vi "Loop_ACT_Drive with Profile.vi"() -> ()   [LabVIEW 2017]
uses:
  _SHARE ALL/Global Share All/Global_STOP.vi
  Global_ACT Write_Data Out.vi
  Global_SM Write_Data Out.vi
  WCDrive2018/WCDrive2018.lvlib
  TypeDef/CLUSTER_Drive_HW_SRX_Status.ctl
  TypeDef/ENUM_Drive_ACT Loop_Mode.ctl
  TypeDef/CLUSTER_X and Y.ctl
  TypeDef/ENUM_Drive_Profile_CMD.ctl
  Dashboard/Global_SEN Write_Data.vi
  TypeDef/CLUSTER_Drive_Point Specification.ctl
  TypeDef/CLUSTER_Drive_Motion Profile Arrays.ctl
  TypeDef/CLUSTER_SRX_Profile Data.ctl
  TypeDef/CLUSTER_SRX_Limit Switch Data.ctl
  TypeDef/CLUSTER_SRX_Analog Data.ctl
  TypeDef/CLUSTER_SRX_PWM Data.ctl
  TypeDef/CLUSTER_SRX_Encoder Data.ctl
  TypeDef/CLUSTER_SRX_Status Data.ctl
  TypeDef/CLUSTER_4296_SRX_Status.ctl
  TypeDef/ENUM_Drive_SRX Motion Buffer Status.ctl
panel:
  out "Output Data":dbl
  out "Input Data":dbl
  out "Cycle Time (S)":dbl format="%.3g"
  in  "Target Time(ms)":u32=50
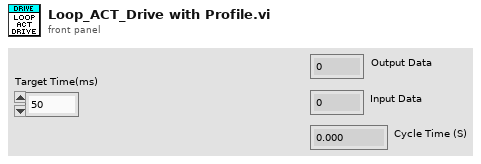
[diagram p1: front panel]
types:
  T1 = typedef "ENUM_Drive_SRX Motion Buffer Status.ctl" = cluster{"Index":i32, "Last Point":bool}
  T2 = typedef "CLUSTER_Drive_Motion Profile Arrays.ctl" = cluster{"Left":T3[], "Right":T3[]}
  T3 = typedef "CLUSTER_Drive_Point Specification.ctl" = cluster{"Position":dbl, "Velocity":dbl, "headingDeg":dbl, "Duration in ms":i32}
  T4 = typedef "ENUM_Drive_Profile_CMD.ctl" = enum16{"Stop", "Setup", "Run"}
  T5 = typedef "CLUSTER_X and Y.ctl" = cluster{"Steer":dbl, "Throtle":dbl}
  T6 = typedef "ENUM_Drive_ACT Loop_Mode.ctl" = enum16{"Stop", "Position", "VBus", "Profile"}
  T7 = typedef "CLUSTER_Drive_HW_SRX_Status.ctl" = cluster{"Rear Left":T8, "Rear Right":T8, "Front Left":T8, "Front Right":T8}
  T8 = typedef "CLUSTER_4296_SRX_Status.ctl" = cluster{"Status":T9, "Encoder":T10, "PWM ":T11, "Analog":T12, "Limit Switches":T13, "Profile":T14}
  T9 = typedef "CLUSTER_SRX_Status Data.ctl" = cluster{"Module Enabled":bool, "Current Profile Slot Select":dbl, "Brake is Enabled":bool, "Applied Throttle":dbl, "Current":dbl, "Battery Voltage":dbl, "Sticky Fault - Under Voltage":bool, "Temperature (C)":dbl, "Sticky Fault - Over Temp":bool, "CAN Error":errorcluster, "Control 5 Is Supported":bool}
  T10 = typedef "CLUSTER_SRX_Encoder Data.ctl" = cluster{"Closed Loop Error":dbl, "Sensor Position":dbl, "Sensor Velocity":dbl, "Encoder Position":dbl, "Encoder Velocity":dbl, "Encoder Index Count":dbl, "Encoder A Pin State":bool, "Encoder B Pin State":bool, "Encoder Index Pin State":bool, "Pos Div 8":bool, "Vel Div 4":bool}
  T11 = typedef "CLUSTER_SRX_PWM Data.ctl" = cluster{"Closed Loop Error":dbl, "Pulse Width Position":i32, "Pulse Width Velocity":i32, "Pulse Width Rise To Rise (us)":i32, "Pulse Width Rise To Fall (us)":i32}
  T12 = typedef "CLUSTER_SRX_Analog Data.ctl" = cluster{"Closed Loop Error":dbl, "Analog In":dbl, "Analog In Velocity":dbl}
  T13 = typedef "CLUSTER_SRX_Limit Switch Data.ctl" = cluster{"Forward Limit Switch Closed":bool, "Reverse Limit Switch Closed":bool, "Sticky Fault - Forward Limit":bool, "Sticky Fault - Reverse Limit":bool, "Sticky Fault - Forward Soft Limit":bool, "Sticky Fault - Reverse Soft Limit":bool}
  T14 = typedef "CLUSTER_SRX_Profile Data.ctl" = cluster{"Mot Prof Active Is Under Run":bool, "Mot Prof Active Has Under Run":bool, "Mot Prof Active Is Last":bool, "Mot Prof Active Velocity Only":bool, "Mot Prof Active Is Valid":bool, "Mot Prof Buffer Is Full":bool, "Mot Prof Active Profile Slot Select":i32, "Mot Prof NextID":i32, "Mot Prof Count":i32, "Mot Prof Active Velocity":dbl, "Mot Prof Active Position":dbl, "Mot Prof Output Enable":i32}
  T15 = typedef "WPI_RobotDriveDevRef.ctl" = cluster{"DevStatus":errorcluster, "Motors[]":T16[], "Square Inputs":bool, "Max Output":dbl}
  T16 = typedef "WPI_MotorControlDeviceRef.ctl" = cluster{"DeviceStatus":errorcluster, "Type":T17, "PWM":cluster{"PWM Channel":T18, "DeadBand":T19}, "CAN":cluster{"Device Number":u8, "SetOutput VI Ref":variant, "GetOutput VI Ref":variant, "Enable VI Ref":variant, "Disable VI Ref":variant, "Data":variant}, "Invert":bool, "DIO PWM":cluster{"PWM \"Enable\" Channel":T18, "DIOChannel":T20, "PWM Rate":dbl}}
  T17 = typedef "WPI_MotorControlType.ctl" = enum16{"PWM", "CAN", "DIO PWM"}
  T18 = typedef "FPGA_DIOPWMChannel.ctl" = enum8{"PWM 0", "PWM 1", "PWM 2", "PWM 3", "PWM 4", "PWM 5", "PWM 6", "PWM 7", "PWM 8", "PWM 9", "PWM MXP 0", "PWM MXP 1", "PWM MXP 2", "PWM MXP 3", "PWM MXP 4", "PWM MXP 5", "PWM MXP 6", "PWM MXP 7", "PWM MXP 8", "PWM MXP 9", "Invalid"}
  T19 = typedef "WPI_PWMDeadband.ctl" = cluster{"Name":string, "maxPositivePwm":i32, "minPositivePwm":i32, "centerPwm":i32, "maxNegativePwm":i32, "minNegativePwm":i32, "angularRange":u16}
  T20 = typedef "FPGA_DIOChannel.ctl" = enum8{"DIO 0", "DIO 1", "DIO 2", "DIO 3", "DIO 4", "DIO 5", "DIO 6", "DIO 7", "DIO 8", "DIO 9", "DIO MXP 0", "DIO MXP 1", "DIO MXP 2", "DIO MXP 3", "DIO MXP 4", "DIO MXP 5", "DIO MXP 6", "DIO MXP 7", "DIO MXP 8", "DIO MXP 9", "DIO MXP 10", "DIO MXP 11", "DIO MXP 12", "DIO MXP 13", "DIO MXP 14", "DIO MXP 15", "SPI Port CS1", "SPI Port CS2", "SPI Port CS3", "SPI Port MISO", "SPI Port MOSI", "Invalid"}
  T21 = cluster{"RobotDriveDevRef Out":T15, "Target Time(ms)":u32, "Current Time":timestamp, "Previous Time":timestamp, "Cycle Time (S)":dbl, "SRX_Status":T7, "Mode":T6, "VBus":T5, "ProfileCmd":T4, "MotionProfiles":T2, "Buffer Status Array":T1[]}
  T22 = typedef "CLUSTER_Left and Right.ctl" = cluster{"Left":dbl, "Right":dbl}
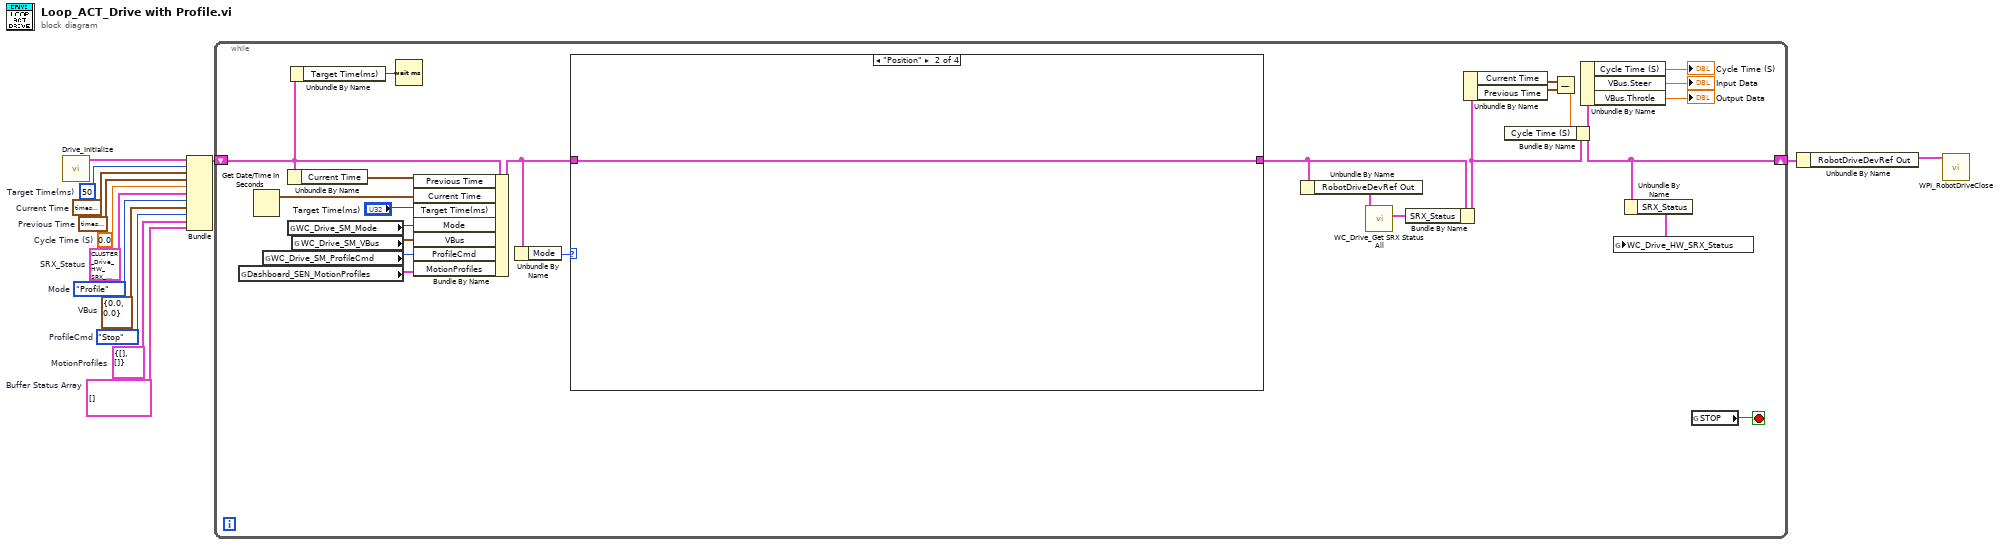
[diagram p0: block diagram]
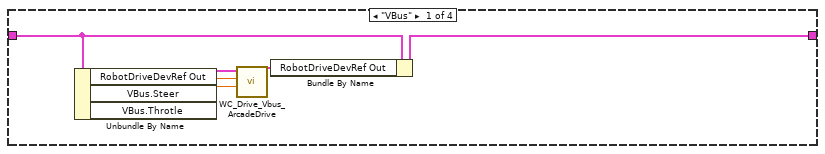
[diagram p2: hidden frame]
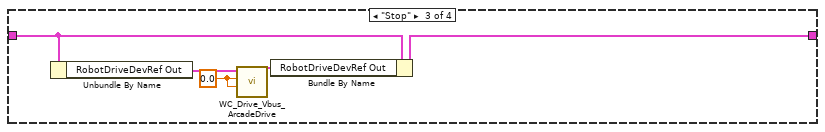
[diagram p3: hidden frame]
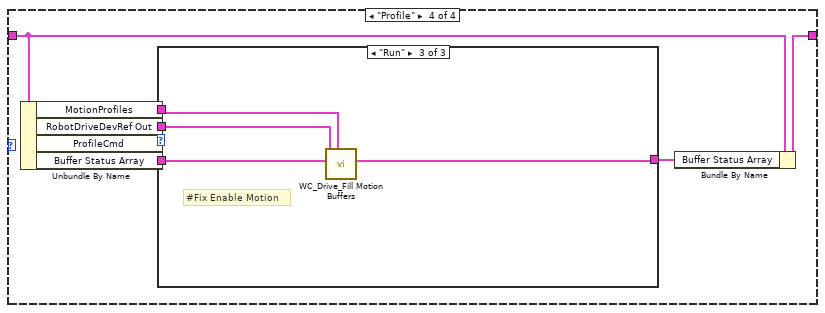
[diagram p4: hidden frame]
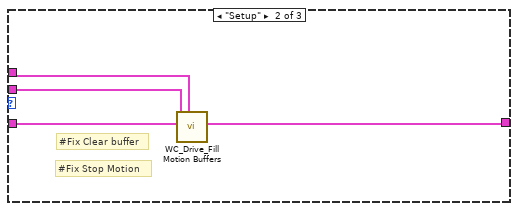
[diagram p6: hidden frame]
diagram:
  w1 = T1[] []  # Buffer Status Array
  w2 = T2 {"Left"=[], "Right"=[]}  # MotionProfiles
  w3 = ENUM_Drive_Profile_CMD."Stop"  # ProfileCmd
  w4 = T5 {"Steer"=0.0, "Throtle"=0.0}  # VBus
  w5 = ENUM_Drive_ACT_Loop_Mode."Profile"  # Mode
  w6 = T7 {"Rear Left"={"Status"={"Module Enabled"=FALSE, "Current Profile Slot Select"=0.0, "Brake is Enabled"=FALSE, "Applied Throttle"=0.0, "Current"=0.0, "Battery Voltage"=0.0, "Sticky Fault - Under Voltage"=FALSE, "Temperature (C)"=0.0, "Sticky Fault - Over Temp"=FALSE, "CAN Error"={"status"=FALSE, "code"=0, "source"=""}, "Control 5 Is Supported"=FALSE}, "Encoder"={"Closed Loop Error"=0.0, "Sensor Position"=0.0, "Sensor Velocity"=0.0, "Encoder Position"=0.0, "Encoder Velocity"=0.0, "Encoder Index Count"=0.0, "Encoder A Pin State"=FALSE, "Encoder B Pin State"=FALSE, "Encoder Index Pin State"=FALSE, "Pos Div 8"=FALSE, "Vel Div 4"=FALSE}, "PWM "={"Closed Loop Error"=0.0, "Pulse Width Position"=0, "Pulse Width Velocity"=0, "Pulse Width Rise To Rise (us)"=0, "Pulse Width Rise To Fall (us)"=0}, "Analog"={"Closed Loop Error"=0.0, "Analog In"=0.0, "Analog In Velocity"=0.0}, "Limit Switches"={"Forward Limit Switch Closed"=FALSE, "Reverse Limit Switch Closed"=FALSE, "Sticky Fault - Forward Limit"=FALSE, "Sticky Fault - Reverse Limit"=FALSE, "Sticky Fault - Forward Soft Limit"=FALSE, "Sticky Fault - Reverse Soft Limit"=FALSE}, "Profile"={"Mot Prof Active Is Under Run"=FALSE, "Mot Prof Active Has Under Run"=FALSE, "Mot Prof Active Is Last"=FALSE, "Mot Prof Active Velocity Only"=FALSE, "Mot Prof Active Is Valid"=FALSE, "Mot Prof Buffer Is Full"=FALSE, "Mot Prof Active Profile Slot Select"=0, "Mot Prof NextID"=0, "Mot Prof Count"=0, "Mot Prof Active Velocity"=0.0, "Mot Prof Active Position"=0.0, "Mot Prof Output Enable"=0}}, "Rear Right"={"Status"={"Module Enabled"=FALSE, "Current Profile Slot Select"=0.0, "Brake is Enabled"=FALSE, "Applied Throttle"=0.0, "Current"=0.0, "Battery Voltage"=0.0, "Sticky Fault - Under Voltage"=FALSE, "Temperature (C)"=0.0, "Sticky Fault - Over Temp"=FALSE, "CAN Error"={"status"=FALSE, "code"=0, "source"=""}, "Control 5 Is Supported"=FALSE}, "Encoder"={"Closed Loop Error"=0.0, "Sensor Position"=0.0, "Sensor Velocity"=0.0, "Encoder Position"=0.0, "Encoder Velocity"=0.0, "Encoder Index Count"=0.0, "Encoder A Pin State"=FALSE, "Encoder B Pin State"=FALSE, "Encoder Index Pin State"=FALSE, "Pos Div 8"=FALSE, "Vel Div 4"=FALSE}, "PWM "={"Closed Loop Error"=0.0, "Pulse Width Position"=0, "Pulse Width Velocity"=0, "Pulse Width Rise To Rise (us)"=0, "Pulse Width Rise To Fall (us)"=0}, "Analog"={"Closed Loop Error"=0.0, "Analog In"=0.0, "Analog In Velocity"=0.0}, "Limit Switches"={"Forward Limit Switch Closed"=FALSE, "Reverse Limit Switch Closed"=FALSE, "Sticky Fault - Forward Limit"=FALSE, "Sticky Fault - Reverse Limit"=FALSE, "Sticky Fault - Forward Soft Limit"=FALSE, "Sticky Fault - Reverse Soft Limit"=FALSE}, "Profile"={"Mot Prof Active Is Under Run"=FALSE, "Mot Prof Active Has Under Run"=FALSE, "Mot Prof Active Is Last"=FALSE, "Mot Prof Active Velocity Only"=FALSE, "Mot Prof Active Is Valid"=FALSE, "Mot Prof Buffer Is Full"=FALSE, "Mot Prof Active Profile Slot Select"=0, "Mot Prof NextID"=0, "Mot Prof Count"=0, "Mot Prof Active Velocity"=0.0, "Mot Prof Active Position"=0.0, "Mot Prof Output Enable"=0}}, "Front Left"={"Status"={"Module Enabled"=FALSE, "Current Profile Slot Select"=0.0, "Brake is Enabled"=FALSE, "Applied Throttle"=0.0, "Current"=0.0, "Battery Voltage"=0.0, "Sticky Fault - Under Voltage"=FALSE, "Temperature (C)"=0.0, "Sticky Fault - Over Temp"=FALSE, "CAN Error"={"status"=FALSE, "code"=0, "source"=""}, "Control 5 Is Supported"=FALSE}, "Encoder"={"Closed Loop Error"=0.0, "Sensor Position"=0.0, "Sensor Velocity"=0.0, "Encoder Position"=0.0, "Encoder Velocity"=0.0, "Encoder Index Count"=0.0, "Encoder A Pin State"=FALSE, "Encoder B Pin State"=FALSE, "Encoder Index Pin State"=FALSE, "Pos Div 8"=FALSE, "Vel Div 4"=FALSE}, "PWM "={"Closed Loop Error"=0.0, "Pulse Width Position"=0, "Pulse Width Velocity"=0, "Pulse Width Rise To Rise (us)"=0, "Pulse Width Rise To Fall (us)"=0}, "Analog"={"Closed Loop Error"=0.0, "Analog In"=0.0, "Analog In Velocity"=0.0}, "Limit Switches"={"Forward Limit Switch Closed"=FALSE, "Reverse Limit Switch Closed"=FALSE, "Sticky Fault - Forward Limit"=FALSE, "Sticky Fault - Reverse Limit"=FALSE, "Sticky Fault - Forward Soft Limit"=FALSE, "Sticky Fault - Reverse Soft Limit"=FALSE}, "Profile"={"Mot Prof Active Is Under Run"=FALSE, "Mot Prof Active Has Under Run"=FALSE, "Mot Prof Active Is Last"=FALSE, "Mot Prof Active Velocity Only"=FALSE, "Mot Prof Active Is Valid"=FALSE, "Mot Prof Buffer Is Full"=FALSE, "Mot Prof Active Profile Slot Select"=0, "Mot Prof NextID"=0, "Mot Prof Count"=0, "Mot Prof Active Velocity"=0.0, "Mot Prof Active Position"=0.0, "Mot Prof Output Enable"=0}}, "Front Right"={"Status"={"Module Enabled"=FALSE, "Current Profile Slot Select"=0.0, "Brake is Enabled"=FALSE, "Applied Throttle"=0.0, "Current"=0.0, "Battery Voltage"=0.0, "Sticky Fault - Under Voltage"=FALSE, "Temperature (C)"=0.0, "Sticky Fault - Over Temp"=FALSE, "CAN Error"={"status"=FALSE, "code"=0, "source"=""}, "Control 5 Is Supported"=FALSE}, "Encoder"={"Closed Loop Error"=0.0, "Sensor Position"=0.0, "Sensor Velocity"=0.0, "Encoder Position"=0.0, "Encoder Velocity"=0.0, "Encoder Index Count"=0.0, "Encoder A Pin State"=FALSE, "Encoder B Pin State"=FALSE, "Encoder Index Pin State"=FALSE, "Pos Div 8"=FALSE, "Vel Div 4"=FALSE}, "PWM "={"Closed Loop Error"=0.0, "Pulse Width Position"=0, "Pulse Width Velocity"=0, "Pulse Width Rise To Rise (us)"=0, "Pulse Width Rise To Fall (us)"=0}, "Analog"={"Closed Loop Error"=0.0, "Analog In"=0.0, "Analog In Velocity"=0.0}, "Limit Switches"={"Forward Limit Switch Closed"=FALSE, "Reverse Limit Switch Closed"=FALSE, "Sticky Fault - Forward Limit"=FALSE, "Sticky Fault - Reverse Limit"=FALSE, "Sticky Fault - Forward Soft Limit"=FALSE, "Sticky Fault - Reverse Soft Limit"=FALSE}, "Profile"={"Mot Prof Active Is Under Run"=FALSE, "Mot Prof Active Has Under Run"=FALSE, "Mot Prof Active Is Last"=FALSE, "Mot Prof Active Velocity Only"=FALSE, "Mot Prof Active Is Valid"=FALSE, "Mot Prof Buffer Is Full"=FALSE, "Mot Prof Active Profile Slot Select"=0, "Mot Prof NextID"=0, "Mot Prof Count"=0, "Mot Prof Active Velocity"=0.0, "Mot Prof Active Position"=0.0, "Mot Prof Output Enable"=0}}}  # SRX_Status
  w9 = 0.0  # Cycle Time (S)
  w14 = timestamp(0 s since 1904-01-01)  # Previous Time
  w13 = timestamp(0 s since 1904-01-01)  # Current Time
  w12 = u32 50  # Target Time(ms)
  n1 = call "Drive_Initialize.vi"() -> ("RobotDriveDevRef Out"=w8:T15)  [unwired: 11 in]
  n2 = Bundle("RobotDriveDevRef Out"=w8, "Target Time(ms)"=w12, "Current Time"=w13, "Previous Time"=w14, "Cycle Time (S)"=w9, "SRX_Status"=w6, "Mode"=w5, "VBus"=w4, "ProfileCmd"=w3, "MotionProfiles"=w2, "Buffer Status Array"=w1) -> (w11:T21)  [unwired: 1 in]
  n3 = while {
    shift-right: [w22] -> w10
    shift-left: w11 -> [w18]
    stop <- w38 stop-if-true
    n4 = global read "Global_SEN Write_Data.vi" "Dashboard_SEN_MotionProfiles"() -> (w16:T2)
    n5 = Get Date/Time In Seconds() -> (seconds since 1Jan1904=w37:timestamp)
    n6 = global read "Global_SM Write_Data Out.vi" "WC_Drive_SM_ProfileCmd"() -> (w19:T4)
    n7 = Unbundle By Name(w18) -> ("Current Time"=w36:timestamp)
    n8 = global read "Global_SM Write_Data Out.vi" "WC_Drive_SM_Mode"() -> (w27:T6)
    n9 = Unbundle By Name(w18) -> ("Target Time(ms)"=w32:u32)
    n10 = global read "Global_SM Write_Data Out.vi" "WC_Drive_SM_VBus"() -> (w26:T22)
    n11 = Wait (ms)(milliseconds to wait=w32) -> ()  [unwired: 1 out]
    n12 = Bundle By Name(cluster=w18, "Previous Time"=w36, "Current Time"=w37, "Target Time(ms)"="Target Time(ms)", "Mode"=w27, "VBus"=w26, "ProfileCmd"=w19, "MotionProfiles"=w16) -> (w25:T21)
    n13 = Unbundle By Name(w25) -> ("Mode"=w24:T6)
    n14 = case shown="\"Position\"" w24 {
      tunnel: w25 -> [w40 w45 w48 w53]
      tunnel: [w39 w45 w47 w52] -> w20
      frame "VBus" {
        n15 = Unbundle By Name(w40) -> ("RobotDriveDevRef Out"=w44:T15, "VBus.Steer"=w43:dbl, "VBus.Throtle"=w42:dbl)
        n16 = call "WC_Drive_Vbus_ArcadeDrive.vi"("Right Value"=w42, "Left Value"=w43, "RobotDriveDevRef"=w44) -> ("RobotDriveDevRef Out"=w41:T15)  [unwired: 7 in, 1 out]
        n17 = Bundle By Name(cluster=w40, "RobotDriveDevRef Out"=w41) -> (w39:T21)
      }
      frame "Position" {
      }
      frame "Stop" {
        w46 = 0.0 ("X axis value")
        n18 = Unbundle By Name(w48) -> ("RobotDriveDevRef Out"=w50:T15)
        n19 = call "WC_Drive_Vbus_ArcadeDrive.vi"("Right Value"=w46, "Left Value"=w46, "RobotDriveDevRef"=w50) -> ("RobotDriveDevRef Out"=w49:T15)  [unwired: 7 in, 1 out]
        n20 = Bundle By Name(cluster=w48, "RobotDriveDevRef Out"=w49) -> (w47:T21)
      }
      frame "Profile" {
        n21 = Unbundle By Name(w53) -> ("MotionProfiles"=w55:T2, "RobotDriveDevRef Out"=w56:T15, "ProfileCmd"=w57:T4, "Buffer Status Array"=w54:T1[])
        n22 = case shown="\"Run\"" w57 {
          tunnel: w56 -> [_ w59 w63]
          tunnel: w55 -> [_ w60 w64]
          tunnel: w54 -> [w58 w62 w66]
          tunnel: [w58 w61 w65] -> w51
          frame "Stop" {
            # "#Fix Disable Motion"
          }
          frame "Setup" {
            # "#Fix Stop Motion"
            # "#Fix Clear buffer"
            n23 = call "WC_Drive_Fill Motion Buffers.vi"("MotionProfiles"=w60, "Buffer Status Array"=w62, "RobotDriveDevRef"=w59) -> ("Buffer Status Array Out"=w61:T1[])  [unwired: 5 in, 3 out]
          }
          frame "Run" {
            # "#Fix Enable Motion"
            n24 = call "WC_Drive_Fill Motion Buffers.vi"("MotionProfiles"=w64, "Buffer Status Array"=w66, "RobotDriveDevRef"=w63) -> ("Buffer Status Array Out"=w65:T1[])  [unwired: 5 in, 3 out]
          }
        }
        n25 = Bundle By Name(cluster=w53, "Buffer Status Array"=w51) -> (w52:T21)
      }
    }
    n26 = Unbundle By Name(w20) -> ("RobotDriveDevRef Out"=w17:T15)
    n27 = call "WC_Drive_Get SRX Status All.vi"("WC DevRef"=w17) -> ("WC_Drive_SRX Status Out"=w15:T7)  [unwired: 8 in, 2 out]
    n28 = Bundle By Name(cluster=w20, "SRX_Status"=w15) -> (w21:T21)
    n29 = Unbundle By Name(w21) -> ("Current Time"=w35:timestamp, "Previous Time"=w34:timestamp)
    n30 = Subtract(x=w35, y=w34) -> (x-y=w23:dbl)
    n31 = Bundle By Name(cluster=w21, "Cycle Time (S)"=w23) -> (w22:T21)
    n32 = Unbundle By Name(w22) -> ("Cycle Time (S)"=→"Cycle Time (S)":dbl, "VBus.Steer"=→"Input Data":dbl, "VBus.Throtle"=→"Output Data":dbl)
    n33 = Unbundle By Name(w22) -> ("SRX_Status"=w28:T7)
    n34 = global write "Global_ACT Write_Data Out.vi" "WC_Drive_HW_SRX_Status"(w28) -> ()
    n35 = global read "Global_STOP.vi" "STOP"() -> (w38:bool)
  }
  n36 = Unbundle By Name(w10) -> ("RobotDriveDevRef Out"=w7:T15)
  n37 = call <vilib>:"WPI_RobotDriveClose.vi"("RobotDriveDevRef"=w7) -> ()  [unwired: 10 in, 1 out]
